vi "Read FFT Measurement IQ Amplitudes.vi"(8 "error in (no error)":errorcluster, 9 "Signal (I)":i32(ring) items=["I", "Q"], 10 "Instance (1)":i32=1, 11 "VISA resource name":refnum<visa-resource-name>) -> (0 "error out":errorcluster, 1 "Amplitude":dbl[](array[numeric]) format="%^.3e", 2 "Reliability":i32, 3 "VISA resource name out":refnum<visa-resource-name>)   [LabVIEW 2015, in "Rohde&Schwarz CMXP GPRF.lvlib"]
doc: "Starts a new single shot measurement and returns the measured normalized I adn Q amplitudes in time domain.\n\nAttributes:\nRSCMXPGPRF_ATTR_READ_FFT_MEASUREMENT_IQ_AMPLITUDES_I\nRSCMXPGPRF_ATTR_READ_FFT_MEASUREMENT_IQ_AMPLITUDES_Q\n\nRemote-control commands:\nREAD:GPRF:MEAS<i>:FFTSanalyzer:I?\nREAD:GPRF:MEAS<i>:FFTSanalyzer:Q?"
uses:
  <instrlib>/Rohde&Schwarz CMXP GPRF/Rohde&Schwarz CMXP GPRF.lvlib
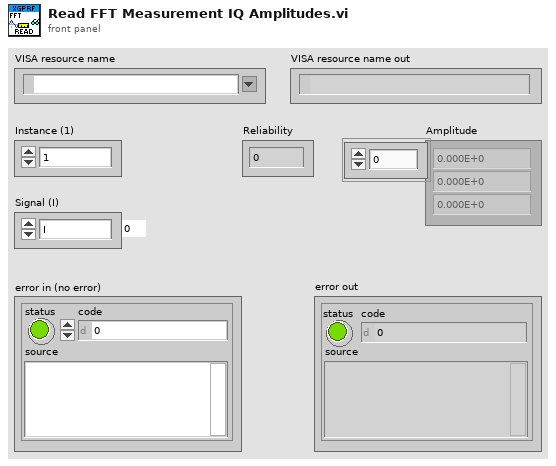
[diagram p1: front panel]
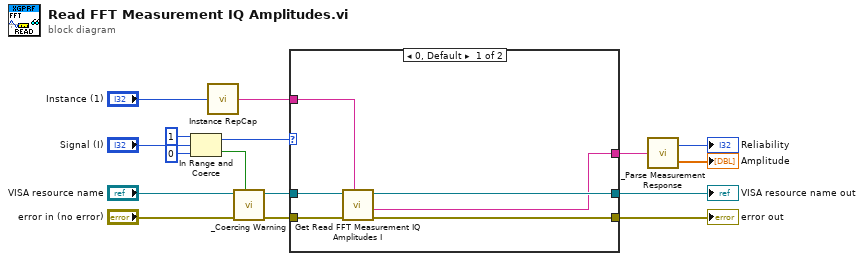
[diagram p0: block diagram]
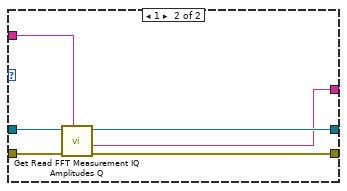
[diagram p2: hidden frame]
diagram:
  n1 = In Range and Coerce(upper limit=1, x="Signal (I)", lower limit=0) -> (coerced(x)=w11:i32, In Range?=w5:bool)
  n2 = call <instrlib>:"Instance RepCap.vi"("instance  in"="Instance (1)") -> ("instance out"=w6:string)
  n3 = call <instrlib>:"_Coercing Warning.vi"("In Range?"=w5, "error in (no error)"="error in (no error)", "VISA resource name"="VISA resource name") -> ("error out"=w10:errorcluster, "VISA resource name out"=w9:refnum<visa-resource-name>)  [unwired: 7 in]
  n4 = case shown="0, Default" w11 {
    tunnel: w10 -> [w22 w28]
    tunnel: w9 -> [w21 w27]
    tunnel: [w20 w26] -> w8
    tunnel: [w19 w25] -> w7
    tunnel: w6 -> [w18 w24]
    tunnel: [w17 w23] -> w3
    frame 0, Default {
      n5 = call "Get Read FFT Measurement IQ Amplitudes I"("Repeated Capabilities"=w18, "error in (no error)"=w22, "instrument handle"=w21) -> ("error out"=w20:errorcluster, "Read FFT Measurement IQ Amplitudes I"=w17:string, "instrument handle out"=w19:refnum<visa-resource-name>)  [unwired: 6 in]
    }
    frame 1 {
      n6 = call "Get Read FFT Measurement IQ Amplitudes Q"("Repeated Capabilities"=w24, "error in (no error)"=w28, "instrument handle"=w27) -> ("error out"=w26:errorcluster, "Read FFT Measurement IQ Amplitudes Q"=w23:string, "instrument handle out"=w25:refnum<visa-resource-name>)  [unwired: 6 in]
    }
  }
  "error out" <- w8
  "VISA resource name out" <- w7
  n7 = call <instrlib>:"_Parse Measurement Response.vi"("String In"=w3) -> ("Reliability"=→"Reliability":i32, "Data"=→"Amplitude":dbl[])
